vi "DirettorePlay.vi"(0 "FPGAReference":refnum<k20>, 1 "NumberOfMatrices":i32, 5 "MatricesArray":i16[](array[numeric]), 7 "DeltaTimeArray":i32[](array[numeric]), 9 "NumberOfTimePointsToPlayArray":i32[](array[numeric]), 11 "SyncArray":i32[](array[numeric])) -> (4 "SpaceLeftInQueue":u32, 15 "ErrorOut":errorcluster)   [LabVIEW 2012]
uses:
  <vilib>/Utility/error.llb/Error Cluster From Error Code.vi
  <vilib>/rvi/errors/niLvFpgaAdjustHostInterfaceError.vi
  <vilib>/rvi/interface/nirviMethod/nirviMethod.xnode
  <vilib>/FPGAPlugInAG/Dynamic/niLvFpga_WriteFifo_Dynamic.vi
  <vilib>/rvi/errors/niLvFpgaMergeErrorWithErrorCode.vi
  <vilib>/FPGAPlugInAG/Dynamic/niLvFpga_ReadFifo_Dynamic.vi
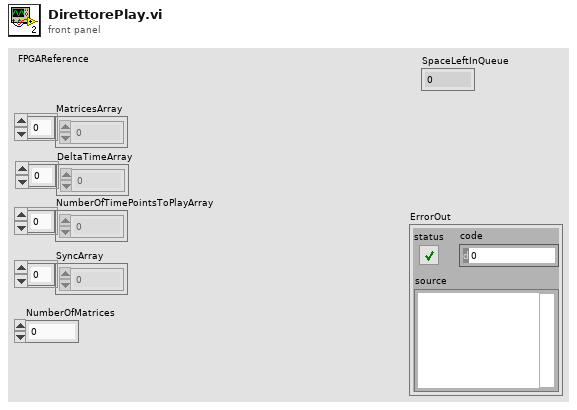
[diagram p1: front panel]
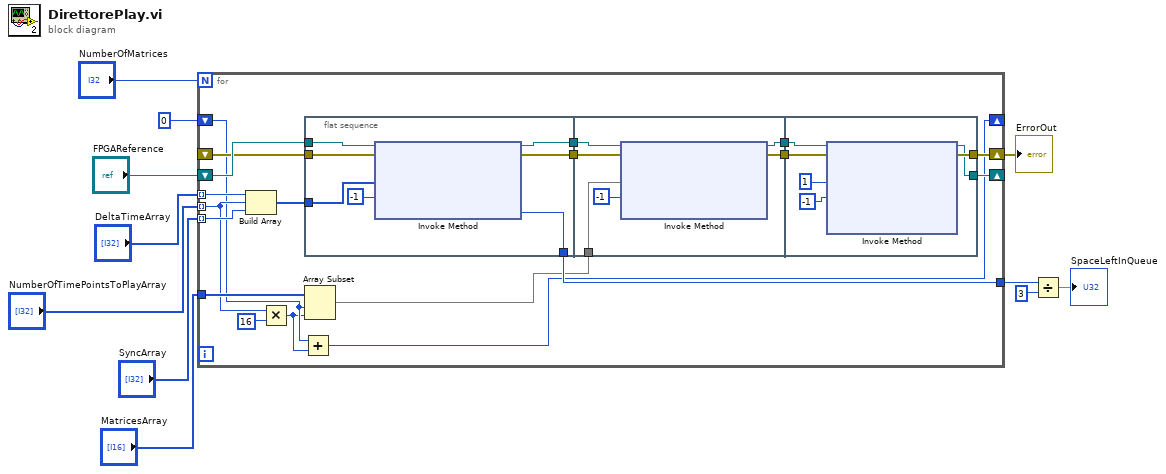
[diagram p0: block diagram]
diagram:
  n1 = for {
    N: "NumberOfMatrices" -> [_]
    shift-right: [w28] -> _
    shift-left: "FPGAReference" -> [w30]
    shift-right: [w27] -> w11
    shift-left: _ -> [w29]
    tunnel: "SyncArray" -> [w22] mode=indexing
    tunnel: "DeltaTimeArray" -> [w23] mode=indexing
    tunnel: [w21] -> w5
    tunnel: "NumberOfTimePointsToPlayArray" -> [w18] mode=indexing
    tunnel: "MatricesArray" -> [w19]
    shift-right: [w15] -> _
    shift-left: 0 ("index") -> [w16]
    n2 = Build Array(w23, w18, w22) -> (w26:i32[])
    n3 = Multiply(x=w18, y=16) -> (x*y=w14:i32)
    n4 = Add(x=w16, y=w14) -> (x+y=w15:i32)
    n5 = flat-sequence {
      tunnel: w30 -> [w36]
      tunnel: w29 -> [w35]
      tunnel: w26 -> [w34]
      tunnel: [w33] -> w25
      tunnel: [w32] -> w24
      tunnel: [w31] -> w21
      tunnel: w20 -> [w40]
      tunnel: w25 -> [w39]
      tunnel: w24 -> [w38]
      tunnel: [w42] -> w13
      tunnel: [w41] -> w12
      tunnel: [w48] -> w27
      tunnel: [w47] -> w28
      tunnel: w13 -> [w46]
      tunnel: w12 -> [w49]
      frame #0 {
        n6 = xnode "Invoke Method"("FPGA VI Reference In"=w36, "error in"=w35, "Data"=w34, "Timeout (ms)"=-1) -> ("FPGA VI Reference Out"=w33:refnum<k20>, "error out"=w32:errorcluster, "Empty Elements Remaining"=w31:u32)
      }
      frame #1 {
        n7 = xnode "Invoke Method"("FPGA VI Reference In"=w39, "error in"=w38, "Data"=w40, "Timeout (ms)"=-1) -> ("FPGA VI Reference Out"=w42:refnum<k20>, "error out"=w41:errorcluster)  [unwired: 1 out]
      }
      frame #2 {
        n8 = xnode "Invoke Method"("FPGA VI Reference In"=w46, "error in"=w49, "Number of Elements"=u32 1, "Timeout (ms)"=-1) -> ("FPGA VI Reference Out"=w47:refnum<k20>, "error out"=w48:errorcluster)  [unwired: 2 out]
      }
    }
    n9 = Array Subset(array=w19, index=w16, length=w14) -> (w20:i16[])
  }
  "ErrorOut" <- w11
  n10 = Divide(x=w5, y=u32 3) -> (x/y=→"SpaceLeftInQueue":dbl)
